vi "Pause.vi"(7 "action":T1, 8 "error in":errorcluster, 10 "Pause!":bool) -> (0 "error out":errorcluster, 2 "Pause?":bool)   [LabVIEW 2018]
uses:
  type defines/Pause action.ctl
  Controls/Queue Manager Actions.ctl
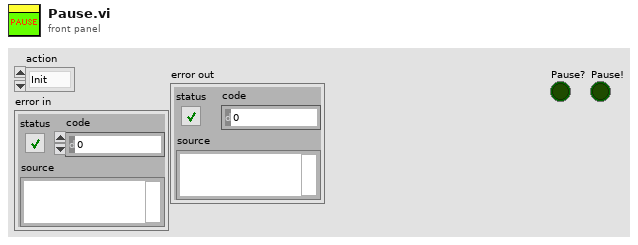
[diagram p1: front panel]
types:
  T1 = typedef "Pause action.ctl" = enum16{"Init", "get", "set"}
  T2 = typedef "Queue Manager Actions.ctl" = enum16{"Init", "Enqueue", "Enqueue All", "Preview Queue", "Dequeue", "Get Status", "Flush Queue", "Flush All Queues", "Release All Queues", "Release Queue", "Enqueue at Opposite End"}
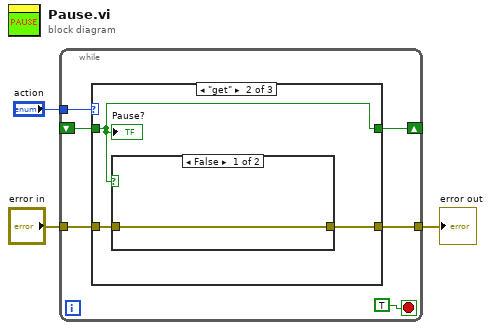
[diagram p0: block diagram]
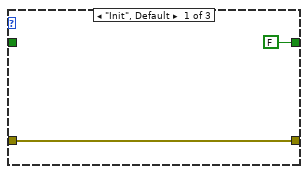
[diagram p2: hidden frame]
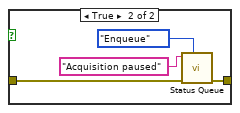
[diagram p3: hidden frame]
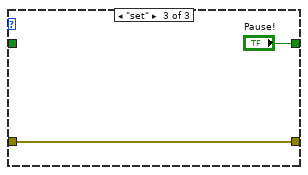
[diagram p4: hidden frame]
diagram:
  n1 = while {
    tunnel: "action" -> [w8]
    shift-right: [w7] -> _
    shift-left: _ -> [w6]
    tunnel: "error in" -> [w5]
    tunnel: [w4] -> w1
    stop <- TRUE stop-if-true
    n2 = case shown="\"get\"" w8 {
      tunnel: [FALSE w12 "Pause!"] -> w7
      tunnel: w6 -> [_ w12 _]
      tunnel: w5 -> [w10 w14 w20]
      tunnel: [w10 w13 w20] -> w4
      frame "Init", Default {
      }
      frame "get" {
        n3 = case shown="False" w12 {
          tunnel: w14 -> [w15 w17]
          tunnel: [w15 w16] -> w13
          frame False {
          }
          frame True {
            n4 = call "Status Queue.vi"("Action"=Queue_Manager_Actions."Enqueue", "Error In"=w17, "Status Message [In]"="Acquisition paused") -> ("Error Out"=w16:errorcluster)  [unwired: 7 in, 1 out]
          }
        }
        "Pause?" <- w12
      }
      frame "set" {
      }
    }
  }
  "error out" <- w1
